vi "Keep true until....vi"(1 "Changer":bool, 2 "Keep":bool) -> (0 "Value":bool)   [LabVIEW 2012]
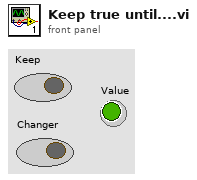
[diagram p1: front panel]
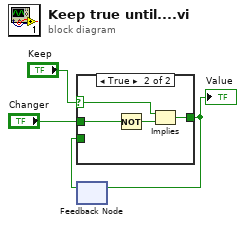
[diagram p0: block diagram]
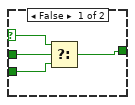
[diagram p2: hidden frame]
diagram:
  n1 = feedback #1() -> (w1:bool)  [unwired: 1 in]
  n2 = case shown="True" "Keep" {
    selector: "Keep" -> [w5 w12]
    tunnel: [w8 w9] -> w2
    tunnel: "Changer" -> [w7 w11]
    tunnel: w1 -> [w6 _]
    frame False {
      n3 = Select(t=w5, s=w7, f=w6) -> (s? t:f=w8:bool)
    }
    frame True {
      n4 = Not(x=w11) -> (.not. x?=w10:bool)
      n5 = Implies(1:w10, 2:w12) -> (0:w9:bool)
    }
  }
  "Value" <- w2
  n6 = feedback-in #1(w2) -> ()
